vi "run.vi"(8 "results reporter":refnum<class "results reporter.lvclass">, 9 "execution system":T1=enum."standard", 10 "thread pool":refnum<class "thread pool.lvclass">, 11 "communicator task in":refnum<class "communicator task.lvclass">) -> (2 "result":refnum<class "result.lvclass">, 3 "communicator task out":refnum<class "communicator task.lvclass">)   [LabVIEW 2015, in "communicator task.lvclass"]
uses:
  communicator task.lvclass
  taskpool/result/result.lvclass
  taskpool/dispatcher/thread pool.lvclass
  taskpool/dispatcher/execution system.ctl
  taskpool/results reporter/results reporter.lvclass
  communicator task.lvclass/communicator task.ctl
  communicator/communicator.lvclass/communicator.ctl
  communicator queue/identifying queue.lvclass
  communicator/communicator.lvclass
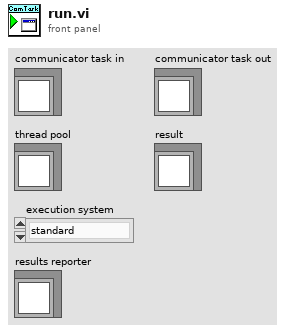
[diagram p1: front panel]
types:
  T1 = typedef "thread pool.lvclass/execution system.ctl" = enum32{"user interface", "standard", "instrument i/o", "data acquisition", "other 1", "other 2"}
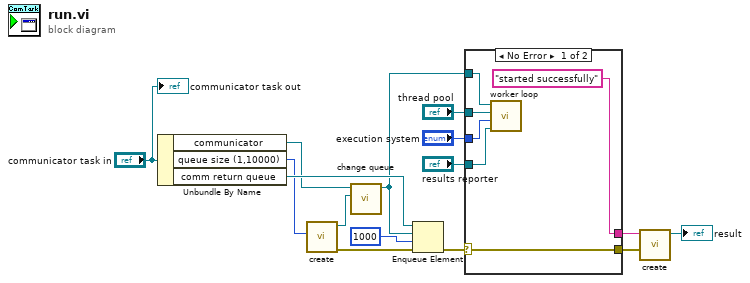
[diagram p0: block diagram]
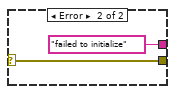
[diagram p2: hidden frame]
diagram:
  n1 = Unbundle By Name("communicator task in") -> ("communicator"=w8:refnum<class "communicator.lvclass">, "queue size (1,10000)"=w9:i32, "comm return queue"=w10:refnum<queue>)
  n2 = call "create.vi"("size (1,10000)"=w9) -> ("error out"=w12:errorcluster, "message connection out"=w6:refnum<class "identifying queue.lvclass">)  [unwired: 9 in]
  n3 = call "change queue.vi"("queue"=w6, "communicator in"=w8) -> ("communicator out"=w7:refnum<class "communicator.lvclass">)  [unwired: 9 in]
  n4 = Enqueue Element(queue=w10, element=w7, timeout in ms (-1)=1000, error in (no error)=w12) -> (error out=w11:errorcluster)  [unwired: 2 out]
  n5 = case shown="No Error" w11 {
    selector: w11 -> [w20 w23]
    tunnel: w7 -> [w21 _]
    tunnel: [w20 w23] -> w5
    tunnel: ["started successfully" "failed to initialize"] -> w4
    tunnel: "thread pool" -> [w18 _]
    tunnel: "execution system" -> [w17 _]
    tunnel: "results reporter" -> [w16 _]
    frame No Error {
      n6 = call "worker loop.vi"("results reporter"=w16, "execution system"=w17, "thread pool"=w18, "communicator in"=w21) -> ()  [unwired: 8 in]
    }
    frame Error {
    }
  }
  n7 = call "create.vi"("error"=w5, "data ID"=w4) -> ("result out"=→"result":refnum<class "result.lvclass">)  [unwired: 9 in]
  "communicator task out" <- "communicator task in"
